vi "DPA.vi"(0 "System no.":i32=1 min=1 max=4 step=1, 2 "Affected items":string[](array[string]), 3 "Password":string="100", 4 "Parameter no. format \n(Decimal: FALSE)":bool, 5 "error in":errorcluster, 6 "Parameter to reset":i32[](array[numeric]), 7 "Parameter to reset (hex)":u32[](array[numeric]) format="%.0x") -> (14 "Controller error":bool, 19 "error out":errorcluster)   [LabVIEW 2020]
doc: "If password is correct, resets parameters or settings to default values, waits 3000 ms and queries ERR?. It does not overwrite settings in the non-volatile memory. For details, see the specific documentation. If parameter no. is in decimal format, use Parameter to reset input, for hexadecimal parameter numbers use Parameter to reset(hex) input and switch Parameter no. format to TRUE. Do not mix decimal and hex. parameter numbers in one call. If Affected items is an empty array, DPA is sent without item and parameter specification.\n\nC-867, C-887, F-206, M-8X0: If Affected items = empty array, the currently valid values of all parameters affected by the specified password are reset. Parameter no. format is FALSE (num.). Only for GCS syntax version = GCS 2.0 or higher (Check with CSV?.vi. If CSV?.vi is not supported, syntax version is GCS 1.0)."
panel:
  # "If password is correct, resets parameters or settings to default values, waits 3000 ms and queries ERR?. It does not overwrite \nsettings in the non-volatile memory. For details, see the specific documentation. If parameter no. is in decimal\nformat, use \"Parameter to reset\" input, for hexadecimal parameter numbers use \"Parameter to reset (hex)\" input and switch \n\"Parameter no. format\" to TRUE.  Do not mix decimal and hex. parameter numbers in one call. If \"Affected items\" is an empty array, \nDPA is sent without item and parameter specification."
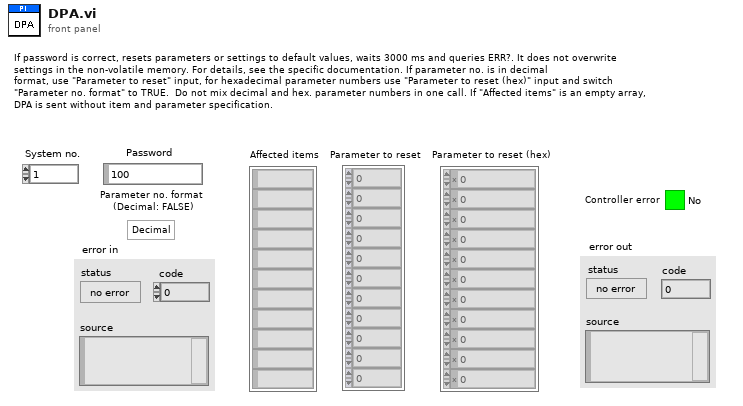
[diagram p1: front panel]
types:
  T1 = enum16{"Disable error check", "Force error check", "Use global settings"}
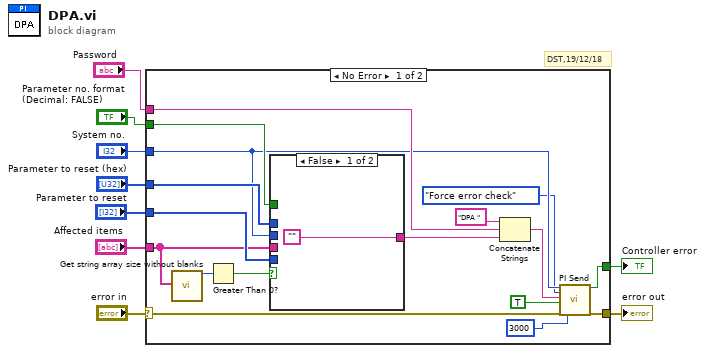
[diagram p0: block diagram]
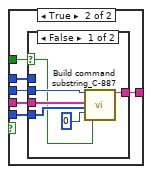
[diagram p2: hidden frame]
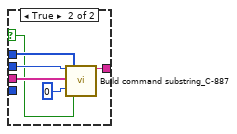
[diagram p3: hidden frame]
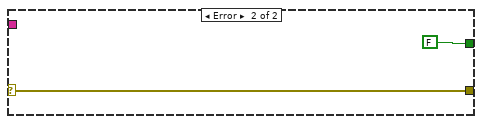
[diagram p4: hidden frame]
diagram:
  # "DST,19/12/18"
  n1 = case shown="No Error" "error in" {
    selector: "error in" -> [w13 w46]
    tunnel: [w10 w46] -> w9
    tunnel: "System no." -> [w16 _]
    tunnel: "Password" -> [w24 _]
    tunnel: [w11 FALSE ("Controller error")] -> w7
    tunnel: "Affected items" -> [w22 _]
    tunnel: "Parameter to reset" -> [w23 _]
    tunnel: "Parameter to reset (hex)" -> [w18 _]
    tunnel: "Parameter no. format \n(Decimal: FALSE)" -> [w17 _]
    frame No Error {
      n2 = call "Get string array size without blanks.vi"("String array"=w22) -> ("Corrected array size"=w21:i32)  [unwired: 18 out]
      n3 = Greater Than 0?(x=w21) -> (x > 0?=w20:bool)
      n4 = case shown="False" w20 {
        tunnel: w22 -> [_ w33]
        tunnel: w23 -> [_ w32]
        tunnel: ["" ("Command substring") w31] -> w19
        tunnel: w18 -> [_ w29]
        tunnel: w17 -> [_ w30]
        tunnel: w16 -> [_ w28]
        frame False {
        }
        frame True {
          n5 = case shown="False" w30 {
            selector: w30 -> [w34 w40]
            tunnel: w33 -> [w38 w44]
            tunnel: w32 -> [w37 _]
            tunnel: [w36 w43] -> w31
            tunnel: w29 -> [_ w42]
            tunnel: w28 -> [w35 w41]
            frame False {
              n6 = call "Build command substring_C-887.vi"("System no."=w35, "Affected axes"=w38, "Parameters"=w37, "No. of digits"=i16 0, "Parameter no. format \n(Decimal: FALSE)"=w34) -> ("Command substring"=w36:string)  [unwired: 2 in, 12 out]
            }
            frame True {
              n7 = call "Build command substring_C-887.vi"("System no."=w41, "Affected axes"=w44, "No. of digits"=i16 0, "Parameters (hex)"=w42, "Parameter no. format \n(Decimal: FALSE)"=w40) -> ("Command substring"=w43:string)  [unwired: 2 in, 12 out]
            }
          }
        }
      }
      n8 = Concatenate Strings("DPA ", w24, w19) -> (w25:string)
      n9 = call "PI Send.vi"("System no."=w16, "Error check settings"=T1."Force error check", "String to send"=w25, "Attach termination char.?"=TRUE ("Attach Linefeed?"), "error in"=w13, "Delay before error check (ms)"=u32 3000 ("millisecond timer value")) -> ("Controller error"=w11:bool, "error out"=w10:errorcluster)  [unwired: 12 out]
    }
    frame Error {
    }
  }
  "error out" <- w9
  "Controller error" <- w7
